vi "LS_372_set_zone_properties.vi"() -> ()   [LabVIEW 2019]
uses:
  Global/Global Variables/Data_Display_global.vi
  Instrument_Setup.vi
  Equipment/Lake Shore 372/Lake Shore 372.lvlib
panel:
  out "HeaterZone Tuning Table.txt":string caption="PID Table"
  in  "Pfad zu Heater Table highT":path=path "D:/Software/CryoTUM-develop/sub_vi-s/Heater Tables/HeaterTableLS372_HT.txt"
  out "Pfad zu Heater Table Low T":path=path "D:/Software/CryoTUM-develop/sub_vi-s/Heater Tables/HeaterTableLS372_TT.txt"
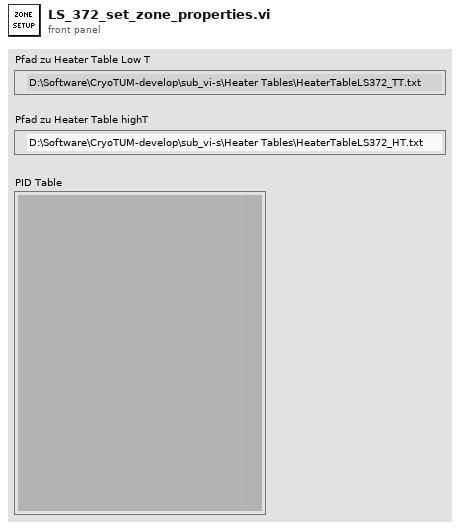
[diagram p1: front panel]
types:
  T1 = enum16{"open", "replace", "create", "open or create", "replace or create", "replace or create with confirmation"}
  T2 = typedef "LS372-Cluster.ctl" = cluster{"Activate Tsweep":bool, "Setpoint - Manual":dbl, "Rate (K/min)":dbl, "Update Lakeshores":bool, "Still Heater":bool, "Still Power (mW)":dbl, "Manual Heater":bool, "Manual Heater  (mW) ":dbl, "Heater Range":dbl, "P (Gain)":dbl, "I (Reset)":dbl, "D (Rate)":dbl, "Heater Power (mW)":dbl, "MC Thermometer":u16, "MC Temperature":dbl, "LS372-T1":dbl, "LS372 -T2":dbl, "LS372-R1 ":dbl, "LS372-R2":dbl, "LS372-T3":dbl, "LS372-T4":dbl, "LS372-R3 ":dbl, "LS372-R4 \n\n\n\n":dbl, "LS372-T5":dbl, "LS372-T6":dbl, "LS372-R5":dbl, "LS372-R6 ":dbl, "Still Power ist":dbl, "Set Temperatur Sweep main":bool, "Setpoint ist":dbl, "Disable Heater":bool}
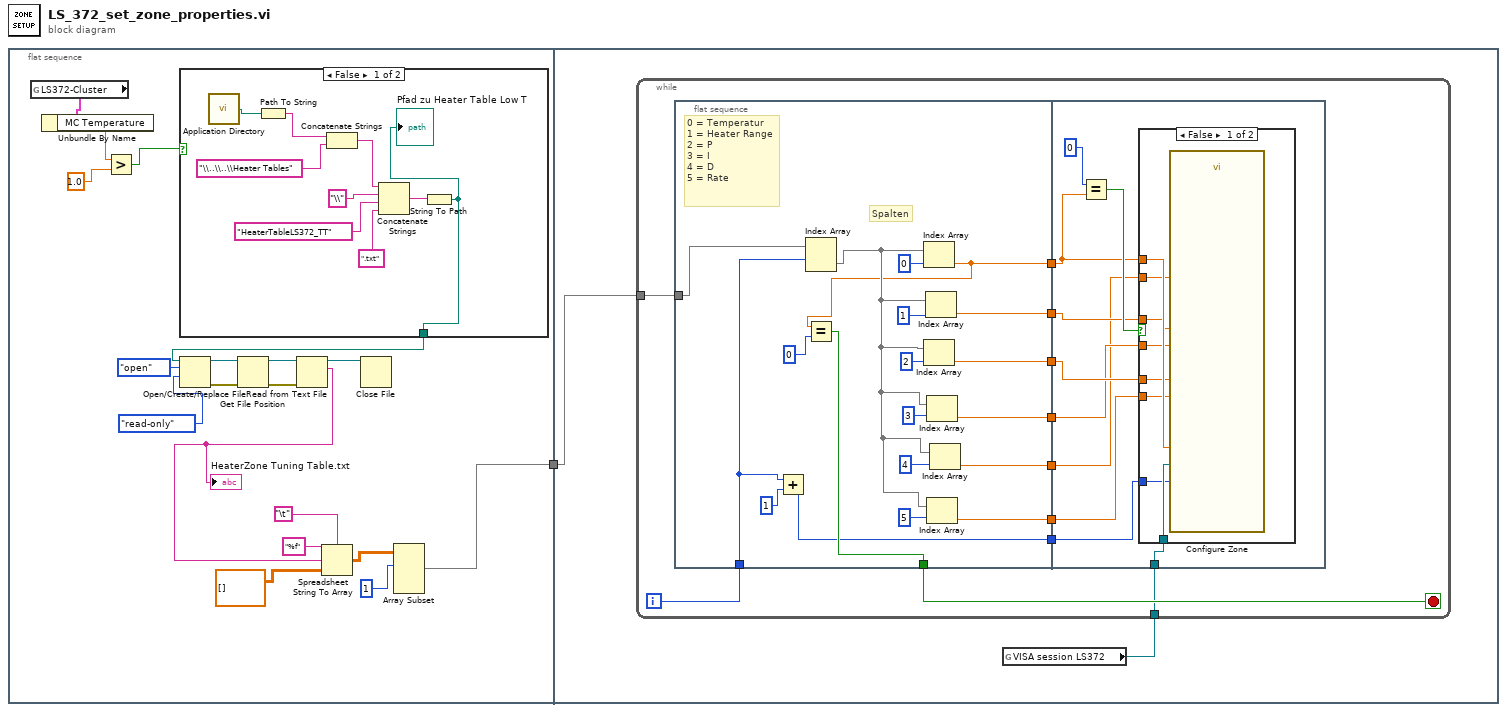
[diagram p0: block diagram]
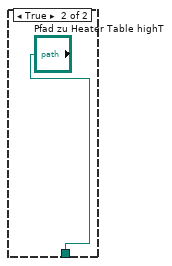
[diagram p2: hidden frame]
diagram:
  n1 = flat-sequence {
    tunnel: [w7] -> w1
    tunnel: w1 -> [w32]
    frame #0 {
      n2 = global read "Data_Display_global.vi" "LS372-Cluster"() -> (w6:T2)
      n3 = Unbundle By Name(w6) -> ("MC Temperature"=w5:dbl)
      n4 = Greater?(x=w5, y=1.0) -> (0:w3:bool)
      n5 = case shown="False" w3 {
        tunnel: [w21 "Pfad zu Heater Table highT"] -> w2
        frame False {
          n6 = call <vilib>:"Application Directory.vi"() -> ("Application Directory"=w29:path)
          n7 = Path To String(path=w29) -> (string=w28:string)
          n8 = Concatenate Strings(w28, "\\..\\..\\Heater Tables") -> (w26:string)
          n9 = Concatenate Strings(w26, "\\", "HeaterTableLS372_TT", ".txt") -> (w22:string)
          n10 = String To Path(string=w22) -> (path=w21:path)
          "Pfad zu Heater Table Low T" <- w21
        }
        frame True {
        }
      }
      n11 = Open/Create/Replace File(file path (use dialog)=w2, operation (0:open)=T1."open", access (0:read/write)=enum16{"read/write", "read-only", "write-only"}."read-only") -> (refnum out=w19:refnum<file>, error out=w20:errorcluster)  [unwired: 3 in, 1 out]
      n12 = Get File Position(4:w20, 7:w19) -> (0:w18:errorcluster, 3:w17:refnum<file>)  [unwired: 1 out]
      n13 = Read from Text File(file (use dialog)=w17, error in=w18) -> (refnum out=w16:refnum<file>, text=w11:string)  [unwired: 2 in, 2 out]
      "HeaterZone Tuning Table.txt" <- w11
      n14 = Spreadsheet String To Array(delimiter (Tab)="\t", format string="%f", spreadsheet string=w11, array type (2D Dbl)=dbl[][] []) -> (array=w9:dbl[][])
      n15 = Close File(refnum=w16) -> ()  [unwired: 1 in, 2 out]
      n16 = Array Subset(array=w9, index (row)=1) -> (w7:dbl[][])  [unwired: 3 in]
    }
    frame #1 {
      n17 = global read "Instrument_Setup.vi" "VISA session LS372"() -> (w31:refnum<visa-resource-name>)
      n18 = while {
        tunnel: w32 -> [w43]
        tunnel: w31 -> [w34]
        i -> [w42]
        stop <- w41 stop-if-true
        n19 = flat-sequence {
          tunnel: w43 -> [w62]
          tunnel: w42 -> [w46]
          tunnel: [w52] -> w41
          tunnel: [w54] -> w40
          tunnel: [w51] -> w39
          tunnel: [w50] -> w38
          tunnel: [w49] -> w37
          tunnel: [w48] -> w36
          tunnel: [w47] -> w35
          tunnel: [w44] -> w33
          tunnel: w40 -> [w70]
          tunnel: w39 -> [w69]
          tunnel: w38 -> [w68]
          tunnel: w37 -> [w67]
          tunnel: w36 -> [w66]
          tunnel: w35 -> [w65]
          tunnel: w34 -> [w64]
          tunnel: w33 -> [w63]
          frame #0 {
            # "0 = Temperatur\n1 = Heater Range\n2 = P\n3 = I\n4 = D\n5 = Rate"
            # "Spalten"
            n20 = Add(x=w46, y=1) -> (x+y=w44:i32)
            n21 = Index Array(array=w62, index (row)=w46) -> (element=w55:dbl[])  [unwired: 1 in]
            n22 = Index Array(array=w55, index=0) -> (element=w54:dbl)
            n23 = Equal?(x=w54, y=0) -> (x = y?=w52:bool)
            n24 = Index Array(array=w55, index=2) -> (element=w50:dbl)
            n25 = Index Array(array=w55, index=1) -> (element=w51:dbl)
            n26 = Index Array(array=w55, index=3) -> (element=w49:dbl)
            n27 = Index Array(array=w55, index=5) -> (element=w47:dbl)
            n28 = Index Array(array=w55, index=4) -> (element=w48:dbl)
          }
          frame #1 {
            n29 = Equal?(x=0, y=w70) -> (x = y?=w71:bool)
            n30 = case shown="False" w71 {
              tunnel: w70 -> [w80 _]
              tunnel: w69 -> [w79 _]
              tunnel: w68 -> [w78 _]
              tunnel: w67 -> [w77 _]
              tunnel: w66 -> [w76 _]
              tunnel: w65 -> [w75 _]
              tunnel: w64 -> [w74 _]
              tunnel: w63 -> [w73 _]
              frame False {
                n31 = call "Configure Zone.vi"("VISA resource name"=w74, "Zone (1)"=w73, "Upper Bound (0.00000E+0)"=w80, "P Value (10.000)"=w78, "Heater Range (0: Off)"=w79, "I Value (20)"=w77, "Ramp Rate (0)"=w75, "D Value (0)"=w76) -> ()  [unwired: 10 in, 2 out]
              }
              frame True {
              }
            }
          }
        }
      }
    }
  }
